vi "Stage_var.vi"() -> ()   [LabVIEW 2019]
panel:
  in  "Stage":u32
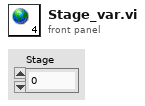
[diagram p1: front panel]
diagram:
